vi "setMagnet.vi"(4 "Mode":T2, 6 "Axis":T1=enum."Z", 8 "error in (no error)":errorcluster, 9 "Target Rate (T/min)":dbl, 10 "Target Field (T)":dbl, 11 "Instrument.VRM in":refnum<class "Instrument.OxfordVRM.lvclass">) -> (0 "error out":errorcluster, 3 "Instrument.VRM out":refnum<class "Instrument.OxfordVRM.lvclass">)   [LabVIEW 2019, in "Instrument.OxfordVRM.lvclass"]
uses:
  Instrument.OxfordVRM.lvclass
  C:/Program Files (x86)/National Instruments/LabVIEW 2019/user.lib/LevyLab/Instrument Framework/Instrument/Instrument.lvclass
  <userlib>/LevyLab/Instrument Framework/Instrument Types/Cryostat/Typedefs/Magnet Mode--Enum.ctl
  <userlib>/LevyLab/Instrument Framework/Instrument Types/Cryostat/Typedefs/Magnet Axis--Enum.ctl
  67c79f1b-78d1-46dd-8fbd-3891f861635a.vi/4df56aec-b636-4272-9157-33732482f91a.vi
  67c79f1b-78d1-46dd-8fbd-3891f861635a.vi/4df56aec-b636-4272-9157-33732482f91a.vi/bcaf770c-9b05-4520-8e7f-bfc2f6a23ddd.vi
  67c79f1b-78d1-46dd-8fbd-3891f861635a.vi/4df56aec-b636-4272-9157-33732482f91a.vi/b050ae4a-267f-4cf6-8c96-46d27b917026.vi
  <userlib>/LevyLab/Instrument Framework/Instrument/API/Remote Client.vi
  <vilib>/Utility/Data Type/Get Type Information.vi
  <vilib>/JDP Science/JSONtext/JSON text to Variant.vi
  <vilib>/JDP Science/JSONtext/LVClass Serializer/JSONtext LVClass Serializer.lvclass
  <userlib>/LevyLab/Instrument Framework/Instrument Types/Cryostat/Instrument.Cryostat.lvclass
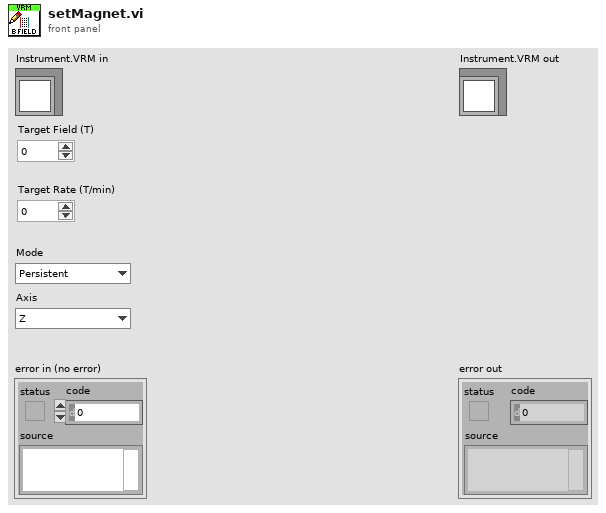
[diagram p1: front panel]
types:
  T1 = typedef "Instrument.Cryostat.lvclass/Magnet Axis--Enum.ctl" = enum16{"X", "Y", "Z"}
  T2 = typedef "Instrument.Cryostat.lvclass/Magnet Mode--Enum.ctl" = enum16{"Persistent", "Driven"}
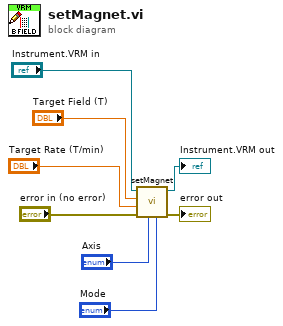
[diagram p0: block diagram]
diagram:
  n1 = call-parent "setMagnet.vi"("Mode"="Mode", "Axis"="Axis", "error in (no error)"="error in (no error)", "Target Rate (T/min)"="Target Rate (T/min)", "Target Field (T)"="Target Field (T)", "Instrument.Cryostat in"="Instrument.VRM in") -> ("error out"=→"error out":errorcluster, "Instrument.Cryostat out"=→"Instrument.VRM out":refnum<class "Instrument.OxfordVRM.lvclass">)  [unwired: 4 in]
